vi "五参数水样测试.vi"(11 "启动参数":T1={"测量模式"=enum."水样测试", "数据类型"="N", "手动启动标记"=FALSE}) -> ()   [LabVIEW 2016, in "斯坦道原位多参数.lvlib"]
panel:
  out "Elapsed Time (s)":dbl caption="已用时间(s)"
  out "状态":string
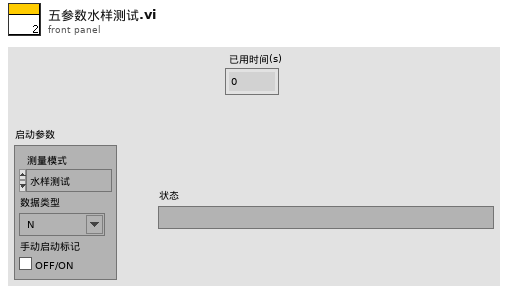
[diagram p1: front panel]
types:
  T1 = typedef "斯坦道原位多参数.lvlib/水样测试启动自定义输入参数.ctl" = cluster{"测量模式":enum16{"待机", "水样测试", "标样核查", "零点核查", "跨度核查", "空白测试", "平行样测试", "加标回收", "空白校准", "标样校准", "初始化（清洗）"}, "数据类型":string, "手动启动标记":bool}
  T2 = cluster{"时间标识":timestamp, "设备":string, "日志信息":string, "流程参数":string}
  T3 = cluster{"水温":bool, "pH":bool, "DO":bool, "DOper":bool, "电导率":bool, "ORP":bool, "浊度":bool, "叶绿素a":bool, "藻密度":bool}
  T4 = cluster{"水样数据时间":timestamp, "检测值":cluster{"水温":dbl, "pH":dbl, "DO":dbl, "DOper":dbl, "电导率":dbl, "ORP":dbl, "浊度":dbl, "叶绿素a":dbl, "藻密度":dbl}}
  T5 = cluster{"系统时间":timestamp, "工作状态":u16, "测量模式":u16, "告警代码":enum16{"无告警", "缺试剂告警", "缺水样告警", "缺蒸馏水告警", "缺标液告警", "仪表漏液告警", "标定异常告警", "超量程告警", "加热异常", "低试剂预警", "超上限告警", "超下限告警", "仪表内部其他异常", "滴定异常告警", "电极异常告警", "量程切换告警", "参数设置告警", "PH电极电位异常", "电导率电极异常", "浊度光度异常", "溶解氧电极异常", "溶解氧光强异常", "温度异常告警", "PH异常告警", "溶解氧异常告警", "电导率异常告警", "浊度异常告警", "叶绿素异常告警", "藻密度异常告警", "蓝绿藻异常告警", "ORP异常告警", "氨氮异常告警", "清洁刷异常告警", "SD卡异常告警", "蓝牙异常告警", "Wifi异常告警", "流程异常告警"}, "故障代码":enum16{"无故障", "电机故障", "温度故障", "通讯故障", "滴定故障"}, "日志代码":u16, "软件版本":string}
  T6 = cluster{"水温":dbl, "pH":dbl, "DO":dbl, "Cond":dbl, "Turb":dbl, "叶绿素":dbl, "藻密度":dbl, "蓝绿藻":dbl, "ORP":dbl, "NH3N":dbl}
  T7 = cluster{"因子编码":string, "单位":string, "标样参考值":sgl, "水样数据时间":timestamp, "水样实测值":sgl, "水样数据标识":string, "K":sgl, "B":sgl, "T":sgl, "H":sgl, "水深":sgl, "探头温度":sgl}
  T8 = enum16{"待机", "水样测试", "标样核查", "零点核查", "跨度核查", "空白测试", "平行样测试", "加标回收", "空白校准", "标样校准", "初始化（清洗）"}
  T9 = cluster{"数据类型":string, "测量模式":enum16{"待机", "水样测试", "标样核查", "零点核查", "跨度核查", "空白测试", "平行样测试", "加标回收", "空白校准", "标样校准", "初始化（清洗）"}}
  T10 = cluster{"测量量程":dbl, "测量精度":dbl, "测量间隔":dbl, "消解温度":dbl, "消解时长":dbl, "空白校准时间":timestamp, "曲线截距":dbl, "曲线斜率":dbl, "测量检出限":dbl, "测量信号值":dbl, "线性相关系数":dbl, "二次多项式系数":dbl, "标样校准时间":timestamp, "稀释倍数":dbl, "三项式系数":dbl, "空白标定系数":dbl, "量程系数":dbl, "F0/ORPA":dbl, "F1/ORPB":dbl, "F2/ORPK":dbl, "F3":dbl, "F4":dbl, "F5":dbl, "F6":dbl, "F7":dbl, "X0/滴定数":dbl, "量程":dbl}
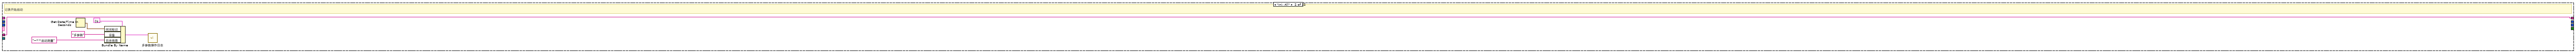
[diagram p3: hidden frame]
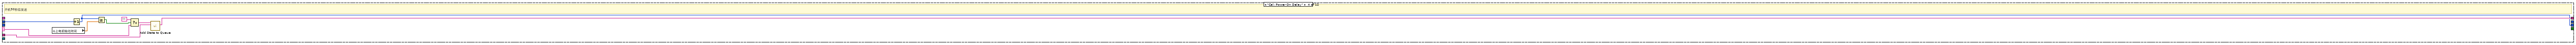
[diagram p5: hidden frame]
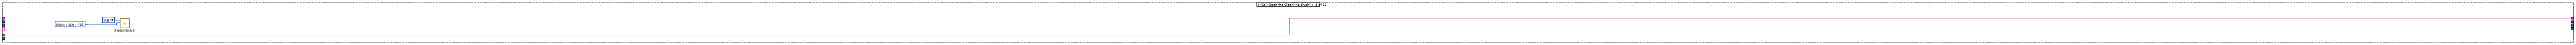
[diagram p6: hidden frame]
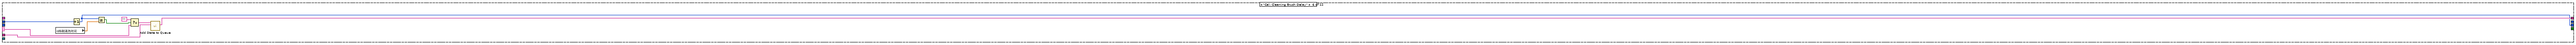
[diagram p7: hidden frame]
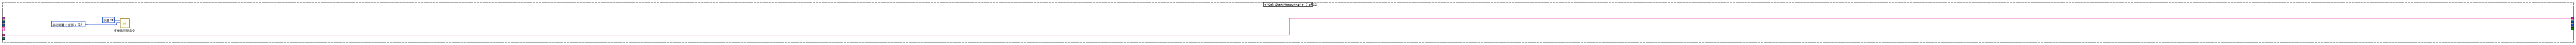
[diagram p8: hidden frame]
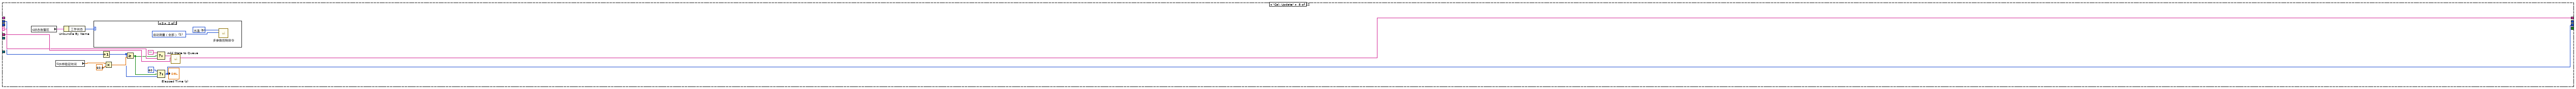
[diagram p9: hidden frame]
diagram:
  w1 = 0  # 存储组数
  n1 = call "Add State to Queue.vi"("State(s) In (\"\")"="Ini: All\nCal: Power On\nCal: Power On Delay\nCal: Open the Cleaning Brush\nCal: Cleaning Brush Delay\nCal: Start Measuring\nCal: Update\nCal: Storing data\nCal: Stop Measuring\nCal: Power Off\nExit" ("State(s) In (\"\")")) -> ("States Out"=w10:string)  [unwired: 14 in]
  n2 = Obtain Notifier(name (unnamed)="MPFlow" ("名称（未命名）"), notification data type=FALSE) -> (notifier out=w4:refnum<notifier>)  [unwired: 2 in, 2 out]
  n3 = Obtain Queue(name (unnamed)="采配水" ("名称（未命名）"), element data type=cluster{"命令":string, "数据":variant} {"命令"="", "数据"=variant}) -> (queue out=w5:refnum<queue>)  [unwired: 3 in, 2 out]
  n4 = while {
    shift-right: [w29] -> _
    shift-left: w10 -> [w31]
    tunnel: w5 -> [w28]
    tunnel: w4 -> [w27]
    tunnel: "启动参数" -> [w26]
    shift-right: [w14] -> _
    shift-left: 0 -> [w15]
    shift-right: [w13] -> _
    shift-left: w1 -> [w12]
    i -> [w24]
    stop <- w22 stop-if-true
    n5 = call "Simple Parse State Queue.vi"("State Queue"=w31) -> ("Remain States"=w30:string, "Next State"=w17:string)  [unwired: 13 in]
    n6 = Wait on Notification(notifier=w27, timeout in ms (-1)=1000 ("超时毫秒(-1)")) -> (notifier out=w21:refnum<notifier>, notification=w19:bool)  [unwired: 2 in, 2 out]
    n7 = Select(t="Exit" ("State(s) In (\"\")"), s=w19, f=w17) -> (s? t:f=w16:string)
    n8 = case shown="\"Cal: Storing data\"" w16 {
      selector: w16 -> [_ _ _ w46 _ w56 _ w74 _ _ _ _]
      tunnel: w30 -> [w32 w38 w39 w48 w51 w60 w61 w75 w87 w399 w408 w411]
      tunnel: [w32 w38 w39 w47 w51 w59 w61 w71 w89 w399 w408 w411] -> w29
      tunnel: w28 -> [_ _ _ _ _ _ _ _ _ _ _ w410]
      tunnel: w21 -> [_ _ _ _ _ _ _ _ _ _ _ w409]
      tunnel: w26 -> [_ _ _ _ _ _ _ _ w95 _ _ _]
      tunnel: [_ _ _ _ _ _ _ _ _ _ _ TRUE] -> w22
      tunnel: w15 -> [_ _ _ w43 _ w55 _ w70 w86 _ _ _]
      tunnel: [_ _ _ w42 _ w54 _ w65 w83 _ _ _] -> w14
      tunnel: w12 -> [_ _ _ _ _ _ _ _ w94 _ _ _]
      tunnel: [_ _ _ _ _ _ _ _ w91 _ _ _] -> w13
      frame Default {
      }
      frame "Ini: All" {
        # "记录开始启动"
        n9 = Get Date/Time In Seconds() -> (seconds since 1Jan1904=w34:timestamp)
        n10 = Bundle By Name(cluster=T2 {"时间标识"=timestamp(0 s since 1904-01-01), "设备"="", "日志信息"="", "流程参数"=""} ("data in"), "时间标识"=w34, "设备"="多参数", "日志信息"="-->>启动测量") -> (w35:T2)
        n11 = call "多参数操作日志.vi"("data in"=w35) -> ()  [unwired: 10 in, 1 out]
      }
      frame "Cal: Power On" {
      }
      frame "Cal: Power On Delay" {
        # "开机30秒后发送"
        n12 = global read "多参数断电保存全局变量.vi" "上电初始化时间"() -> (w40:dbl)
        n13 = Increment(x=w43) -> (x+1=w42:i32)
        n14 = Greater Or Equal?(x=w42, y=w40) -> (x >= y?=w41:bool)
        n15 = Select(t="", s=w41, f=w46) -> (s? t:f=w44:string)
        n16 = call "Add State to Queue.vi"("State(s) In Front (\"\")"=w44, "State(s) In (\"\")"=w48) -> ("States Out"=w47:string)  [unwired: 13 in]
      }
      frame "Cal: Open the Cleanling Brush" {
        w50 = u16 10 items=["启动测量（全部）"=1, "初始化（清洗）"=10, "停止测量（全部）"=11, "校时"=13, "启动测量（单个传感器）"=19, "停止测量（单个传感器）"=20] ("控制命令")
        w49 = u16 9 items=["氨氮"=3, "水温"=9, "pH值"=10, "溶解氧"=11, "电导率"=12, "浊度"=13, "叶绿素a"=14, "藻密度"=15, "蓝绿藻"=16, "氧化还原电位"=17, "溶解氧%"=18, "盐度"=19] ("站号")
        n17 = call "多参数控制命令.vi"("控制命令"=w50, "站号"=w49) -> ()  [unwired: 9 in, 1 out]
      }
      frame "Cal: Cleaning Brush Delay" {
        n18 = global read "多参数断电保存全局变量.vi" "转刷清洗时间"() -> (w52:dbl)
        n19 = Increment(x=w55) -> (x+1=w54:i32)
        n20 = Greater Or Equal?(x=w54, y=w52) -> (x >= y?=w53:bool)
        n21 = Select(t="", s=w53, f=w56) -> (s? t:f=w57:string)
        n22 = call "Add State to Queue.vi"("State(s) In Front (\"\")"=w57, "State(s) In (\"\")"=w60) -> ("States Out"=w59:string)  [unwired: 13 in]
      }
      frame "Cal: Start Measuring" {
        w63 = u16 1 items=["启动测量（全部）"=1, "初始化（清洗）"=10, "停止测量（全部）"=11, "校时"=13, "启动测量（单个传感器）"=19, "停止测量（单个传感器）"=20] ("控制命令")
        w62 = u16 9 items=["氨氮"=3, "水温"=9, "pH值"=10, "溶解氧"=11, "电导率"=12, "浊度"=13, "叶绿素a"=14, "藻密度"=15, "蓝绿藻"=16, "氧化还原电位"=17, "溶解氧%"=18, "盐度"=19] ("站号")
        n23 = call "多参数控制命令.vi"("控制命令"=w63, "站号"=w62) -> ()  [unwired: 9 in, 1 out]
      }
      frame "Cal: Update" {
        n24 = global read "多参数全局变量.vi" "状态告警区"() -> (w77:T5)
        n25 = global read "多参数断电保存全局变量.vi" "水样稳定时间"() -> (w68:dbl)
        n26 = Unbundle By Name(w77) -> ("工作状态"=w78:u16)
        n27 = case shown="0" w78 {
          frame Default {
          }
          frame 0 {
            w79 = u16 1 items=["启动测量（全部）"=1, "初始化（清洗）"=10, "停止测量（全部）"=11, "校时"=13, "启动测量（单个传感器）"=19, "停止测量（单个传感器）"=20] ("控制命令")
            w80 = u16 9 items=["氨氮"=3, "水温"=9, "pH值"=10, "溶解氧"=11, "电导率"=12, "浊度"=13, "叶绿素a"=14, "藻密度"=15, "蓝绿藻"=16, "氧化还原电位"=17, "溶解氧%"=18, "盐度"=19] ("站号")
            n28 = call "多参数控制命令.vi"("控制命令"=w79, "站号"=w80) -> ()  [unwired: 9 in, 1 out]
          }
        }
        n29 = Increment(x=w70) -> (x+1=w66:i32)
        n30 = Multiply(x=w68, y=60.0) -> (x*y=w69:dbl)
        n31 = Greater Or Equal?(x=w66, y=w69) -> (x >= y?=w67:bool)
        n32 = Select(t="", s=w67, f=w74) -> (s? t:f=w73:string)
        n33 = Select(t=60, s=w67, f=w66) -> (s? t:f=w65:i32)
        "Elapsed Time (s)" <- w65
        n34 = call "Add State to Queue.vi"("State(s) In Front (\"\")"=w73, "State(s) In (\"\")"=w75) -> ("States Out"=w71:string)  [unwired: 13 in]
      }
      frame "Cal: Storing data" {
        n35 = Increment(x=w86) -> (x+1=w84:i32)
        n36 = Greater Or Equal?(x=w86, y=60) -> (x >= y?=w81:bool)
        n37 = case shown="真" w81 {
          tunnel: w95 -> [_ w140]
          frame False {
          }
          frame True {
            n38 = Get Date/Time In Seconds() -> (seconds since 1Jan1904=w149:timestamp)
            n39 = Bundle By Name(cluster=T2 {"时间标识"=timestamp(0 s since 1904-01-01), "设备"="", "日志信息"="", "流程参数"=""} ("data in"), "时间标识"=w149, "设备"="多参数", "日志信息"="存储数据") -> (w150:T2)
            n40 = global read "多参数全局变量.vi" "传感器通道号"() -> (w121:T6)
            n41 = call "多参数操作日志.vi"("data in"=w150) -> ()  [unwired: 10 in, 1 out]
            n42 = Unbundle By Name(w121) -> ("水温"=w119:dbl, "pH"=w122:dbl, "DO"=w124:dbl, "Cond"=w126:dbl, "Turb"=w128:dbl, "ORP"=w130:dbl, "叶绿素"=w132:dbl, "藻密度"=w133:dbl)
            n43 = Not Equal To 0?(x=w119) -> (x != 0?=w120:bool)
            n44 = Not Equal To 0?(x=w122) -> (x != 0?=w123:bool)
            n45 = Not Equal To 0?(x=w126) -> (x != 0?=w127:bool)
            n46 = Not Equal To 0?(x=w130) -> (x != 0?=w131:bool)
            n47 = Not Equal To 0?(x=w128) -> (x != 0?=w129:bool)
            n48 = Not Equal To 0?(x=w132) -> (x != 0?=w134:bool)
            n49 = Not Equal To 0?(x=w133) -> (x != 0?=w135:bool)
            n50 = Not Equal To 0?(x=w124) -> (x != 0?=w125:bool)
            n51 = Bundle By Name(cluster=T3 {"水温"=FALSE, "pH"=FALSE, "DO"=FALSE, "DOper"=FALSE, "电导率"=FALSE, "ORP"=FALSE, "浊度"=FALSE, "叶绿素a"=FALSE, "藻密度"=FALSE} ("columns enable"), "水温"=w120, "pH"=w123, "DO"=w125, "DOper"=w125, "电导率"=w127, "ORP"=w131, "浊度"=w129, "叶绿素a"=w134, "藻密度"=w135) -> (w117:T3)
            n52 = for {
              N: 10 -> [_]
              tunnel: [w186] -> w136
              tunnel: w117 -> [w185]
              tunnel: [w185] -> w108
              tunnel: [w159] -> w107
              tunnel: [w158] -> w106
              tunnel: [w157] -> w105
              tunnel: [w160] -> w104
              tunnel: [w156] -> w103
              tunnel: [w164] -> w102
              tunnel: [w161] -> w101
              tunnel: [w162] -> w100
              tunnel: [w163] -> w99
              stop <- w187 stop-if-true
              n53 = global read "多参数全局变量.vi" "spCond数据区"() -> (w169:T7)
              n54 = global read "多参数全局变量.vi" "叶绿素数据区"() -> (w166:T7)
              n55 = global read "多参数全局变量.vi" "藻密度数据区"() -> (w165:T7)
              n56 = global read "多参数全局变量.vi" "DO%数据区"() -> (w170:T7)
              n57 = global read "多参数全局变量.vi" "Turb数据区"() -> (w167:T7)
              n58 = global read "多参数全局变量.vi" "ORP数据区"() -> (w168:T7)
              n59 = global read "多参数全局变量.vi" "水温数据区"() -> (w173:T7)
              n60 = global read "多参数全局变量.vi" "DO数据区"() -> (w171:T7)
              n61 = global read "多参数全局变量.vi" "pH数据区"() -> (w172:T7)
              n62 = Unbundle By Name(w168) -> ("水样实测值"=w178:sgl)
              n63 = Unbundle By Name(w170) -> ("水样实测值"=w180:sgl)
              n64 = Unbundle By Name(w167) -> ("水样实测值"=w177:sgl)
              n65 = Unbundle By Name(w166) -> ("水样实测值"=w176:sgl)
              n66 = Unbundle By Name(w165) -> ("水样实测值"=w175:sgl)
              n67 = Unbundle By Name(w173) -> ("水样实测值"=w183:sgl)
              n68 = Unbundle By Name(w172) -> ("水样实测值"=w182:sgl)
              n69 = Unbundle By Name(w171) -> ("水样实测值"=w181:sgl)
              n70 = Unbundle By Name(w169) -> ("水样实测值"=w179:sgl)
              n71 = Get Date/Time In Seconds() -> (seconds since 1Jan1904=w155:timestamp)
              n72 = Bundle By Name(cluster=w168, "水样数据时间"=w155) -> (w164:T7)
              n73 = Bundle By Name(cluster=w165, "水样数据时间"=w155) -> (w163:T7)
              n74 = Bundle By Name(cluster=w166, "水样数据时间"=w155) -> (w162:T7)
              n75 = Bundle By Name(cluster=w167, "水样数据时间"=w155) -> (w161:T7)
              n76 = Bundle By Name(cluster=w170, "水样数据时间"=w155) -> (w160:T7)
              n77 = Bundle By Name(cluster=w173, "水样数据时间"=w155) -> (w159:T7)
              n78 = Bundle By Name(cluster=w172, "水样数据时间"=w155) -> (w158:T7)
              n79 = Bundle By Name(cluster=w171, "水样数据时间"=w155) -> (w157:T7)
              n80 = Bundle By Name(cluster=w169, "水样数据时间"=w155) -> (w156:T7)
              n81 = Bundle By Name(cluster=T4 {"水样数据时间"=timestamp(0 s since 1904-01-01), "检测值"={"水温"=0.0, "pH"=0.0, "DO"=0.0, "DOper"=0.0, "电导率"=0.0, "ORP"=0.0, "浊度"=0.0, "叶绿素a"=0.0, "藻密度"=0.0}} ("data in"), "水样数据时间"=w155, "检测值.水温"=w183, "检测值.pH"=w182, "检测值.DO"=w181, "检测值.DOper"=w180, "检测值.电导率"=w179, "检测值.ORP"=w178, "检测值.浊度"=w177, "检测值.叶绿素a"=w176, "检测值.藻密度"=w175) -> (w174:T4)
              n82 = call "多参数数据插入.vi"("columns enable"=w185, "data in"=w174) -> ("error out"=w186:errorcluster)  [unwired: 9 in]
              n83 = Unbundle By Name(w186) -> ("status"=w188:bool)
              n84 = Not(x=w188) -> (.not. x?=w187:bool)
            }
            n85 = Unbundle By Name(w140) -> ("数据类型"=w141:string, "测量模式"=w142:T8, "手动启动标记"=w138:bool)
            n86 = Unbundle By Name(w108) -> ("水温"=w116:bool, "pH"=w115:bool, "DO"=w114:bool, "电导率"=w113:bool, "ORP"=w109:bool, "浊度"=w112:bool, "叶绿素a"=w111:bool, "藻密度"=w110:bool)
            n87 = Bundle("数据类型"=w141, "测量模式"=w142) -> (w143:T9)  [unwired: 1 in]
            n88 = case shown="真" w116 {
              tunnel: w143 -> [w378 w382]
              tunnel: [w378 w382] -> w144
              tunnel: w138 -> [_ w381]
              tunnel: w136 -> [_ _]
              tunnel: w107 -> [_ w379]
              frame False {
              }
              frame True {
                n89 = for {
                  N: 10 -> [_]
                  tunnel: w382 -> [w392]
                  tunnel: w381 -> [w389]
                  tunnel: w379 -> [w383]
                  stop <- w384 stop-if-true
                  n90 = Unbundle By Name(w383) -> ("探头温度"=w385:sgl, "水样数据时间"=w386:timestamp)
                  n91 = Unbundle By Name(w392) -> ("数据类型"=w391:string, "测量模式"=w390:T8)
                  n92 = call "多参数测量数据存储.vi"("数据类型"=w391, "手动启动标记"=w389, "测量模式"=w390, "table输入"="水温", "data in"=w383) -> ("error out"=w388:errorcluster)  [unwired: 6 in]
                  n93 = Unbundle By Name(w388) -> ("status"=w387:bool)
                  n94 = Not(x=w387) -> (.not. x?=w384:bool)
                  n95 = case shown="真" w384 {
                    tunnel: w386 -> [_ w396]
                    tunnel: w385 -> [_ w395]
                    frame False {
                    }
                    frame True {
                      n96 = global read "多参数断电保存全局变量.vi" "水温参数"() -> (w398:T10)
                      n97 = Bundle By Name(cluster=w398, "测量信号值"=w395) -> (w394:T10)
                      n98 = global write "多参数断电保存全局变量.vi" "水温参数"(w394) -> ()
                      n99 = call "关键参数存表.vi"("仪器参数"=w394, "datatime"=w396, "仪器名称"="水温") -> ()  [unwired: 8 in, 1 out]
                    }
                  }
                }
              }
            }
            n100 = case shown="真" w115 {
              tunnel: w144 -> [w346 w351]
              tunnel: [w346 w351] -> w146
              tunnel: w138 -> [_ w349]
              tunnel: w106 -> [_ w347]
              frame False {
              }
              frame True {
                n101 = for {
                  N: 10 -> [_]
                  tunnel: w351 -> [w360]
                  tunnel: w349 -> [w355]
                  stop <- w352 stop-if-true
                  n102 = Unbundle By Name(w360) -> ("数据类型"=w359:string, "测量模式"=w358:T8)
                  n103 = global read "多参数全局变量.vi" "pHmv数据区"() -> (w357:T7)
                  n104 = call "多参数测量数据存储.vi"("数据类型"=w359, "手动启动标记"=w355, "测量模式"=w358, "table输入"="pHmv", "data in"=w357) -> ("error out"=w354:errorcluster)  [unwired: 6 in]
                  n105 = Unbundle By Name(w354) -> ("status"=w353:bool)
                  n106 = Not(x=w353) -> (.not. x?=w352:bool)
                }
                n107 = for {
                  N: 10 -> [_]
                  tunnel: w351 -> [w369]
                  tunnel: w349 -> [w367]
                  tunnel: w347 -> [w364]
                  stop <- w365 stop-if-true
                  n108 = Unbundle By Name(w369) -> ("数据类型"=w371:string, "测量模式"=w370:T8)
                  n109 = call "多参数测量数据存储.vi"("数据类型"=w371, "手动启动标记"=w367, "测量模式"=w370, "table输入"="pH", "data in"=w364) -> ("error out"=w368:errorcluster)  [unwired: 6 in]
                  n110 = Unbundle By Name(w368) -> ("status"=w366:bool)
                  n111 = global read "多参数全局变量.vi" "pHmv数据区"() -> (w363:T7)
                  n112 = Not(x=w366) -> (.not. x?=w365:bool)
                  n113 = Unbundle By Name(w363) -> ("水样实测值"=w361:sgl, "水样数据时间"=w362:timestamp)
                  n114 = case shown="真" w365 {
                    tunnel: w362 -> [_ w375]
                    tunnel: w361 -> [_ w374]
                    frame False {
                    }
                    frame True {
                      n115 = global read "多参数断电保存全局变量.vi" "PH参数"() -> (w377:T10)
                      n116 = Bundle By Name(cluster=w377, "测量信号值"=w374) -> (w373:T10)
                      n117 = global write "多参数断电保存全局变量.vi" "PH参数"(w373) -> ()
                      n118 = call "关键参数存表.vi"("仪器参数"=w373, "datatime"=w375, "仪器名称"="PH") -> ()  [unwired: 8 in, 1 out]
                    }
                  }
                }
              }
            }
            n119 = case shown="真" w114 {
              tunnel: [w313 w321] -> w145
              tunnel: w146 -> [w313 w321]
              tunnel: w138 -> [_ w318]
              tunnel: w105 -> [_ w315]
              tunnel: w104 -> [_ w314]
              frame False {
              }
              frame True {
                n120 = Unbundle By Name(w321) -> ("数据类型"=w319:string, "测量模式"=w320:T8)
                n121 = for {
                  N: 10 -> [_]
                  tunnel: w320 -> [w344]
                  tunnel: w319 -> [w343]
                  tunnel: w318 -> [w342]
                  tunnel: w314 -> [w338]
                  stop <- w339 stop-if-true
                  n122 = call "多参数测量数据存储.vi"("数据类型"=w343, "手动启动标记"=w342, "测量模式"=w344, "table输入"="DO_%", "data in"=w338) -> ("error out"=w341:errorcluster)  [unwired: 6 in]
                  n123 = Unbundle By Name(w341) -> ("status"=w340:bool)
                  n124 = Not(x=w340) -> (.not. x?=w339:bool)
                }
                n125 = for {
                  N: 10 -> [_]
                  tunnel: w320 -> [w331]
                  tunnel: w319 -> [w330]
                  tunnel: w318 -> [w329]
                  tunnel: w315 -> [w323]
                  tunnel: w314 -> [w322]
                  stop <- w326 stop-if-true
                  n126 = Unbundle By Name(w322) -> ("水样实测值"=w324:sgl, "水样数据时间"=w325:timestamp)
                  n127 = call "多参数测量数据存储.vi"("数据类型"=w330, "手动启动标记"=w329, "测量模式"=w331, "table输入"="DO", "data in"=w323) -> ("error out"=w328:errorcluster)  [unwired: 6 in]
                  n128 = Unbundle By Name(w328) -> ("status"=w327:bool)
                  n129 = Not(x=w327) -> (.not. x?=w326:bool)
                  n130 = case shown="真" w326 {
                    tunnel: w325 -> [_ w335]
                    tunnel: w324 -> [_ w334]
                    frame False {
                    }
                    frame True {
                      n131 = global read "多参数断电保存全局变量.vi" "溶解氧参数"() -> (w337:T10)
                      n132 = Bundle By Name(cluster=w337, "测量信号值"=w334) -> (w333:T10)
                      n133 = global write "多参数断电保存全局变量.vi" "溶解氧参数"(w333) -> ()
                      n134 = call "关键参数存表.vi"("仪器参数"=w333, "datatime"=w335, "仪器名称"="溶解氧") -> ()  [unwired: 8 in, 1 out]
                    }
                  }
                }
              }
            }
            n135 = case shown="真" w113 {
              tunnel: w145 -> [w272 w278]
              tunnel: [w272 w278] -> w147
              tunnel: w138 -> [_ w277]
              tunnel: w103 -> [_ w273]
              frame False {
              }
              frame True {
                (unwired) 10
                n136 = for {
                  N: 10 -> [_]
                  tunnel: w278 -> [w287]
                  tunnel: w277 -> [w282]
                  stop <- w279 stop-if-true
                  n137 = Unbundle By Name(w287) -> ("数据类型"=w285:string, "测量模式"=w286:T8)
                  n138 = global read "多参数全局变量.vi" "TDS数据区"() -> (w284:T7)
                  n139 = call "多参数测量数据存储.vi"("数据类型"=w285, "手动启动标记"=w282, "测量模式"=w286, "table输入"="总溶解固体", "data in"=w284) -> ("error out"=w281:errorcluster)  [unwired: 6 in]
                  n140 = Unbundle By Name(w281) -> ("status"=w280:bool)
                  n141 = Not(x=w280) -> (.not. x?=w279:bool)
                }
                n142 = for {
                  N: 10 -> [_]
                  tunnel: w278 -> [w308]
                  tunnel: w277 -> [w307]
                  stop <- w304 stop-if-true
                  n143 = Unbundle By Name(w308) -> ("数据类型"=w310:string, "测量模式"=w309:T8)
                  n144 = global read "多参数全局变量.vi" "Sal数据区"() -> (w312:T7)
                  n145 = call "多参数测量数据存储.vi"("数据类型"=w310, "手动启动标记"=w307, "测量模式"=w309, "table输入"="盐度", "data in"=w312) -> ("error out"=w306:errorcluster)  [unwired: 6 in]
                  n146 = Unbundle By Name(w306) -> ("status"=w305:bool)
                  n147 = Not(x=w305) -> (.not. x?=w304:bool)
                }
                n148 = for {
                  N: 10 -> [_]
                  tunnel: w278 -> [w298]
                  tunnel: w277 -> [w294]
                  tunnel: w273 -> [w288]
                  stop <- w289 stop-if-true
                  n149 = Unbundle By Name(w288) -> ("水样实测值"=w290:sgl, "水样数据时间"=w291:timestamp)
                  n150 = Unbundle By Name(w298) -> ("数据类型"=w297:string, "测量模式"=w296:T8)
                  n151 = call "多参数测量数据存储.vi"("数据类型"=w297, "手动启动标记"=w294, "测量模式"=w296, "table输入"="电导率", "data in"=w288) -> ("error out"=w293:errorcluster)  [unwired: 6 in]
                  n152 = Unbundle By Name(w293) -> ("status"=w292:bool)
                  n153 = Not(x=w292) -> (.not. x?=w289:bool)
                  n154 = case shown="真" w289 {
                    tunnel: w291 -> [_ w301]
                    tunnel: w290 -> [_ w300]
                    frame False {
                    }
                    frame True {
                      n155 = global read "多参数断电保存全局变量.vi" "电导率参数"() -> (w303:T10)
                      n156 = Bundle By Name(cluster=w303, "测量信号值"=w300) -> (w299:T10)
                      n157 = global write "多参数断电保存全局变量.vi" "电导率参数"(w299) -> ()
                      n158 = call "关键参数存表.vi"("仪器参数"=w299, "datatime"=w301, "仪器名称"="电导率") -> ()  [unwired: 8 in, 1 out]
                    }
                  }
                }
              }
            }
            n159 = case shown="真" w112 {
              tunnel: w147 -> [w251 w255]
              tunnel: [w251 w255] -> w153
              tunnel: w138 -> [_ w254]
              tunnel: w101 -> [_ w252]
              frame False {
              }
              frame True {
                n160 = for {
                  N: 10 -> [_]
                  tunnel: w255 -> [w263]
                  tunnel: w254 -> [w262]
                  tunnel: w252 -> [w256]
                  stop <- w257 stop-if-true
                  n161 = Unbundle By Name(w256) -> ("水样实测值"=w258:sgl, "水样数据时间"=w259:timestamp)
                  n162 = Unbundle By Name(w263) -> ("数据类型"=w264:string, "测量模式"=w265:T8)
                  n163 = call "多参数测量数据存储.vi"("数据类型"=w264, "手动启动标记"=w262, "测量模式"=w265, "table输入"="浊度", "data in"=w256) -> ("error out"=w261:errorcluster)  [unwired: 6 in]
                  n164 = Unbundle By Name(w261) -> ("status"=w260:bool)
                  n165 = Not(x=w260) -> (.not. x?=w257:bool)
                  n166 = case shown="真" w257 {
                    tunnel: w259 -> [_ w269]
                    tunnel: w258 -> [_ w268]
                    frame False {
                    }
                    frame True {
                      n167 = global read "多参数断电保存全局变量.vi" "浊度参数"() -> (w271:T10)
                      n168 = Bundle By Name(cluster=w271, "测量信号值"=w268) -> (w267:T10)
                      n169 = global write "多参数断电保存全局变量.vi" "浊度参数"(w267) -> ()
                      n170 = call "关键参数存表.vi"("仪器参数"=w267, "datatime"=w269, "仪器名称"="浊度") -> ()  [unwired: 8 in, 1 out]
                    }
                  }
                }
              }
            }
            n171 = case shown="真" w111 {
              tunnel: w153 -> [w230 w234]
              tunnel: [w230 w234] -> w154
              tunnel: w138 -> [_ w233]
              tunnel: w100 -> [_ w231]
              frame False {
              }
              frame True {
                n172 = for {
                  N: 10 -> [_]
                  tunnel: w234 -> [w242]
                  tunnel: w233 -> [w241]
                  tunnel: w231 -> [w235]
                  stop <- w236 stop-if-true
                  n173 = Unbundle By Name(w235) -> ("水样实测值"=w237:sgl, "水样数据时间"=w238:timestamp)
                  n174 = Unbundle By Name(w242) -> ("数据类型"=w243:string, "测量模式"=w244:T8)
                  n175 = call "多参数测量数据存储.vi"("数据类型"=w243, "手动启动标记"=w241, "测量模式"=w244, "table输入"="叶绿素a", "data in"=w235) -> ("error out"=w240:errorcluster)  [unwired: 6 in]
                  n176 = Unbundle By Name(w240) -> ("status"=w239:bool)
                  n177 = Not(x=w239) -> (.not. x?=w236:bool)
                  n178 = case shown="真" w236 {
                    tunnel: w238 -> [_ w248]
                    tunnel: w237 -> [_ w247]
                    frame False {
                    }
                    frame True {
                      n179 = global read "多参数断电保存全局变量.vi" "叶绿素参数"() -> (w250:T10)
                      n180 = Bundle By Name(cluster=w250, "测量信号值"=w247) -> (w246:T10)
                      n181 = global write "多参数断电保存全局变量.vi" "叶绿素参数"(w246) -> ()
                      n182 = call "关键参数存表.vi"("仪器参数"=w246, "datatime"=w248, "仪器名称"="叶绿素") -> ()  [unwired: 8 in, 1 out]
                    }
                  }
                }
              }
            }
            n183 = case shown="真" w110 {
              tunnel: w154 -> [w209 w213]
              tunnel: [w209 w213] -> w139
              tunnel: w138 -> [_ w212]
              tunnel: w99 -> [_ w210]
              frame False {
              }
              frame True {
                n184 = for {
                  N: 10 -> [_]
                  tunnel: w213 -> [w221]
                  tunnel: w212 -> [w220]
                  tunnel: w210 -> [w214]
                  stop <- w215 stop-if-true
                  n185 = Unbundle By Name(w214) -> ("水样实测值"=w216:sgl, "水样数据时间"=w217:timestamp)
                  n186 = Unbundle By Name(w221) -> ("数据类型"=w222:string, "测量模式"=w223:T8)
                  n187 = call "多参数测量数据存储.vi"("数据类型"=w222, "手动启动标记"=w220, "测量模式"=w223, "table输入"="藻密度", "data in"=w214) -> ("error out"=w219:errorcluster)  [unwired: 6 in]
                  n188 = Unbundle By Name(w219) -> ("status"=w218:bool)
                  n189 = Not(x=w218) -> (.not. x?=w215:bool)
                  n190 = case shown="真" w215 {
                    tunnel: w217 -> [_ w227]
                    tunnel: w216 -> [_ w226]
                    frame False {
                    }
                    frame True {
                      n191 = global read "多参数断电保存全局变量.vi" "藻密度参数"() -> (w229:T10)
                      n192 = Bundle By Name(cluster=w229, "测量信号值"=w226) -> (w225:T10)
                      n193 = global write "多参数断电保存全局变量.vi" "藻密度参数"(w225) -> ()
                      n194 = call "关键参数存表.vi"("仪器参数"=w225, "datatime"=w227, "仪器名称"="藻密度") -> ()  [unwired: 8 in, 1 out]
                    }
                  }
                }
              }
            }
            n195 = case shown="真" w109 {
              tunnel: w139 -> [_ w192]
              tunnel: w138 -> [_ w191]
              tunnel: w102 -> [_ w189]
              frame False {
              }
              frame True {
                n196 = for {
                  N: 10 -> [_]
                  tunnel: w192 -> [w202]
                  tunnel: w191 -> [w199]
                  tunnel: w189 -> [w193]
                  stop <- w194 stop-if-true
                  n197 = Unbundle By Name(w193) -> ("水样实测值"=w195:sgl, "水样数据时间"=w196:timestamp)
                  n198 = Unbundle By Name(w202) -> ("数据类型"=w200:string, "测量模式"=w201:T8)
                  n199 = call "多参数测量数据存储.vi"("数据类型"=w200, "手动启动标记"=w199, "测量模式"=w201, "table输入"="ORP", "data in"=w193) -> ("error out"=w198:errorcluster)  [unwired: 6 in]
                  n200 = Unbundle By Name(w198) -> ("status"=w197:bool)
                  n201 = Not(x=w197) -> (.not. x?=w194:bool)
                  n202 = case shown="真" w194 {
                    tunnel: w196 -> [_ w206]
                    tunnel: w195 -> [_ w205]
                    frame False {
                    }
                    frame True {
                      n203 = global read "多参数断电保存全局变量.vi" "ORP参数"() -> (w208:T10)
                      n204 = Bundle By Name(cluster=w208, "测量信号值"=w205) -> (w204:T10)
                      n205 = global write "多参数断电保存全局变量.vi" "ORP参数"(w204) -> ()
                      n206 = call "关键参数存表.vi"("仪器参数"=w204, "datatime"=w206, "仪器名称"="ORP") -> ()  [unwired: 8 in, 1 out]
                    }
                  }
                }
              }
            }
          }
        }
        n207 = case shown="真" w81 {
          tunnel: w94 -> [w96 w98]
          tunnel: [w96 w97] -> w91
          frame False {
          }
          frame True {
            n208 = Increment(x=w98) -> (x+1=w97:i32)
          }
        }
        n209 = Select(t=0, s=w81, f=w84) -> (s? t:f=w83:i32)
        n210 = call "Add State to Queue.vi"("State(s) In Front (\"\")"="Cal: Storing data" ("State(s) In Front (\"\")"), "State(s) In (\"\")"=w87) -> ("States Out"=w88:string)  [unwired: 13 in]
        n211 = global read "多参数断电保存全局变量.vi" "水样测试组数"() -> (w92:dbl)
        n212 = Greater Or Equal?(x=w91, y=w92) -> (x >= y?=w90:bool)
        n213 = Select(t=w87, s=w90, f=w88) -> (s? t:f=w89:string)
      }
      frame "Cal: Stop Measuring" {
        n214 = flat-sequence {
          frame #0 {
            w405 = u16 11 items=["启动测量（全部）"=1, "初始化（清洗）"=10, "停止测量（全部）"=11, "校时"=13, "启动测量（单个传感器）"=19, "停止测量（单个传感器）"=20] ("控制命令")
            w406 = u16 9 items=["氨氮"=3, "水温"=9, "pH值"=10, "溶解氧"=11, "电导率"=12, "浊度"=13, "叶绿素a"=14, "藻密度"=15, "蓝绿藻"=16, "氧化还原电位"=17, "溶解氧%"=18, "盐度"=19] ("站号")
            n215 = call "多参数控制命令.vi"("控制命令"=w405, "站号"=w406) -> ()  [unwired: 9 in, 1 out]
          }
          frame #1 {
            n216 = Wait (ms)(milliseconds to wait=u32 2000 ("等待时间（毫秒）")) -> ()  [unwired: 1 out]
          }
        }
        n217 = Get Date/Time In Seconds() -> (seconds since 1Jan1904=w402:timestamp)
        n218 = Bundle By Name(cluster=T2 {"时间标识"=timestamp(0 s since 1904-01-01), "设备"="", "日志信息"="", "流程参数"=""} ("data in"), "时间标识"=w402, "设备"="多参数", "日志信息"="-->>停止测量") -> (w401:T2)
        n219 = call "多参数操作日志.vi"("data in"=w401) -> ()  [unwired: 10 in, 1 out]
      }
      frame "Cal: Power Off" {
      }
      frame "Exit" {
        n220 = Release Notifier(notifier=w409) -> ()  [unwired: 2 in, 3 out]
        n221 = Release Queue(queue=w410) -> ()  [unwired: 2 in, 3 out]
      }
    }
    n222 = Format Into String(format string="当前运行状态：%s  累计运行%d秒" ("格式字符串"), w16, w24) -> (resulting string=w23:string)  [unwired: 2 in, 1 out]
    "状态" <- w23
    n223 = global write "多参数全局变量.vi" "运行状态"(w23) -> ()
  }
